vi "Read_service-name.vi"(8 "error in (no error)":errorcluster, 11 "instrument in":refnum<class "instrument.lvclass">) -> (0 "error out":errorcluster, 2 "service name":string, 3 "instrument out":refnum<class "instrument.lvclass">)   [LabVIEW 2018, in "instrument.lvclass"]
doc: "reads the private property \"service name\""
uses:
  instrument.lvclass
  instrument.lvclass/instrument.ctl
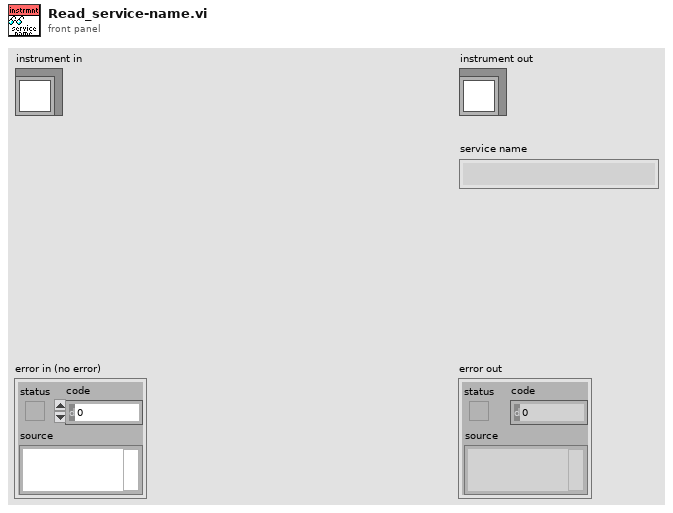
[diagram p1: front panel]
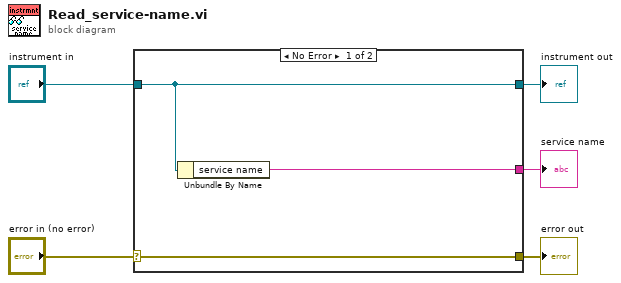
[diagram p0: block diagram]
diagram:
  n1 = case shown="No Error" "error in (no error)" {
    selector: "error in (no error)" -> [w8 w9]
    tunnel: [w8 w9] -> w4
    tunnel: [w7 w10] -> w2
    tunnel: "instrument in" -> [w7 w10]
    tunnel: [w6 _] -> w1
    frame No Error {
      n2 = Unbundle By Name(w7) -> ("service name"=w6:string)
    }
    frame Error {
    }
  }
  "error out" <- w4
  "instrument out" <- w2
  "service name" <- w1
